vi "dfd_Filter Types Are All SOS.vi"(8 "error in (no error)":errorcluster, 11 "filters in":T1[](array[typedef]) {"mSRate_QSettings"."source" items=["Coef a/k"=0, "Coef b/v"=7, "Input"=1, "Output"=2, "Multiplicand"=3, "Product"=4, "Sum"=5, "Delay"=6, "Gain"=8]}) -> (0 "error out":errorcluster, 2 "All SOS?":bool, 3 "filters out":T1[](array[typedef]) {"mSRate_QSettings"."source" items=["Coef a/k"=0, "Coef b/v"=7, "Input"=1, "Output"=2, "Multiplicand"=3, "Product"=4, "Sum"=5, "Delay"=6, "Gain"=8]})   [LabVIEW 2017, in "NI_DigFilterLicensed.lvlib"]
uses:
  <vilib>/addons/Digital Filter Design/NI_DigFilterLicensed.lvlib
  <vilib>/addons/Digital Filter Design/_Objects.llb/DFD Filter Obj.ctl
  <vilib>/addons/Digital Filter Design/_Objects.llb/DFD Filter Coef.ctl
  <vilib>/addons/Digital Filter Design/_Objects.llb/DFD Filter Structure Type Selector.ctl
  <vilib>/addons/Digital Filter Design/_Objects.llb/dfd_Internal Quantization Settings.ctl
  <vilib>/addons/Digital Filter Design/_Objects.llb/dfd_Internal Quantization Srcs.ctl
  <vilib>/addons/Digital Filter Design/_Objects.llb/DFD Coef Norm Type.ctl
  <vilib>/addons/Digital Filter Design/_Objects.llb/DFD Filter Structure Id.ctl
  <vilib>/addons/Digital Filter Design/FilterLib.llb/dfd_Get Filter Coef Type (Filter IO).vi
  <vilib>/addons/Digital Filter Design/_Misc.llb/dfd_Error Handlers (Single).vi
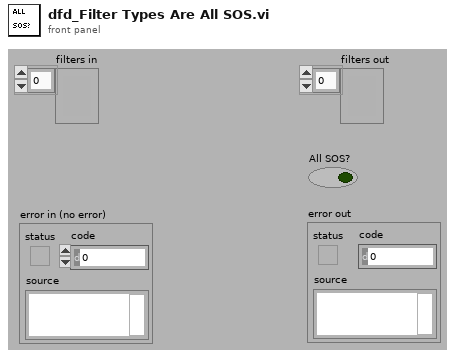
[diagram p1: front panel]
types:
  T1 = typedef "NI_DigFilterLicensed.lvlib/DFD Filter Obj.ctl" = cluster{"mSRate_Fs":dbl, "mSRate_Version":string, "mSRate_Comments":string, "mSRate_OrgCoef":T2, "mSRate_CurCoef":T2, "mSRate_Quantized?":bool, "mSRate_QCoef":T2, "mSRate_QSettings":T4[], "mSRate_Order":i32, "mSRate_Scaling":cluster{"mSRate_ScaleByPowerOf2?":bool, "mSRate_ScaleType":T6}}
  T2 = typedef "NI_DigFilterLicensed.lvlib/DFD Filter Coef.ctl" = cluster{"type":T3, "gain":dbl, "coef a (k)":dbl[], "coef b (v)":dbl[]}
  T3 = typedef "NI_DigFilterLicensed.lvlib/DFD Filter Structure Type Selector.ctl" = enum16{"Undefined", "FIR Direct Form", "FIR Direct Form Transposed", "FIR Symmetric", "FIR Antisymmetric", "IIR Direct Form I", "IIR Direct Form I Transposed", "IIR Direct Form II", "IIR Direct Form II Transposed", "IIR Cascaded Second Order Sections Form I", "IIR Cascaded Second Order Sections Form I Transposed", "IIR Cascaded Second Order Sections Form II", "IIR Cascaded Second Order Sections Form II Transposed", "Lattice Allpass (basic sections)", "Lattice Allpass (one multiplier sections)", "Lattice Allpass (normalized sections)", "Lattice AR (basic sections)", "Lattice AR (one multiplier sections)", "Lattice AR (normalized sections)", "Lattice MA (minimum phase)", "Lattice MA (maximum phase)", "Lattice ARMA (basic sections)", "Lattice ARMA (one multiplier sections)", "Lattice ARMA (normalized sections)"}
  T4 = typedef "NI_DigFilterLicensed.lvlib/dfd_Internal Quantization Settings.ctl" = cluster{"source":T5, "wl":i16, "iwl":i16, "overflow mode":enum16{"Saturation", "Wrap"}, "rounding mode":enum16{"Nearest", "Truncation"}, "signed?":bool}
  T5 = typedef "NI_DigFilterLicensed.lvlib/dfd_Internal Quantization Srcs.ctl" = u16
  T6 = typedef "NI_DigFilterLicensed.lvlib/DFD Coef Norm Type.ctl" = enum16{"No Norm", "Time Domain 1-Norm", "Time Domain 2-Norm", "Time Domain Inf-Norm"}
  T7 = typedef "NI_DigFilterLicensed.lvlib/DFD Filter Structure Id.ctl" = enum16{"Undefined", "FIR", "IIR Direct", "IIR SOS", "IIR Allpass", "IIR AR", "IIR ARMA"}
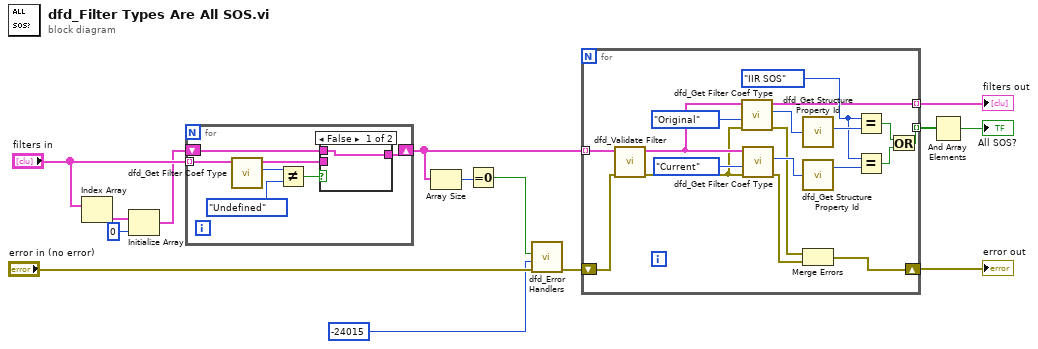
[diagram p0: block diagram]
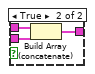
[diagram p2: hidden frame]
diagram:
  n1 = Index Array(array="filters in") -> (element=w8:T1)  [unwired: 1 in]
  n2 = Initialize Array(w8, 0 ("dimension size")) -> (w7:T1[])
  n3 = for {
    shift-right: [w19] -> w6
    shift-left: w7 -> [w18]
    tunnel: "filters in" -> [w17] mode=indexing
    n4 = call-poly <vilib>:"dfd_Get Filter Coef Type.vi"("filter in"=w17) -> ("type"=w21:T3, "filter out"=w16:T1)  [unwired: 2 in, 7 out]
    n5 = Not Equal?(x=w21, y=DFD_Filter_Structure_Type_Selector."Undefined") -> (x != y?=w15:bool)
    n6 = case shown="False" w15 {
      tunnel: [w22 w25] -> w19
      tunnel: w18 -> [w22 w24]
      tunnel: w16 -> [_ w23]
      frame False {
      }
      frame True {
        n7 = Build Array (concatenate)(w24, w23) -> (w25:T1[])
      }
    }
  }
  n8 = Array Size(array=w6) -> (size(s)=w5:i32)
  n9 = Equal To 0?(x=w5) -> (x = 0?=w2:bool)
  n10 = call-poly <vilib>:"dfd_Error Handlers.vi"("error in (no error)"="error in (no error)", "error code"=-24015 ("ERR_INVALID_FILTER_OBJ"), "condition failed?"=w2) -> ("error out"=w3:errorcluster)  [unwired: 8 out]
  n11 = for {
    tunnel: [w34] -> w11 mode=indexing
    shift-right: [w29] -> w14
    shift-left: w3 -> [w26]
    tunnel: [w28] -> w13 mode=indexing
    tunnel: w6 -> [w27] mode=indexing
    w37 = DFD_Filter_Structure_Id."IIR SOS" ("x")
    n12 = call <vilib>:"dfd_Validate Filter.vi"("error in (no error)"=w26, "filter in"=w27) -> ("error out"=w32:errorcluster, "filter out"=w33:T1)  [unwired: 1 in, 7 out]
    n13 = call-poly <vilib>:"dfd_Get Filter Coef Type.vi"("error in (no error)"=w32, "coef source"=enum16{"Original", "Current", "Quantized"}."Original", "filter in"=w33) -> ("error out"=w31:errorcluster, "type"=w41:T3, "filter out"=w28:T1)  [unwired: 6 out]
    n14 = call-poly <vilib>:"dfd_Get Filter Coef Type.vi"("error in (no error)"=w32, "coef source"=enum16{"Original", "Current", "Quantized"}."Current", "filter in"=w33) -> ("error out"=w30:errorcluster, "type"=w40:T3)  [unwired: 7 out]
    n15 = call <vilib>:"dfd_Get Structure Property Id.vi"("structure type"=w41) -> ("filter structure id"=w39:T7)  [unwired: 1 out]
    n16 = call <vilib>:"dfd_Get Structure Property Id.vi"("structure type"=w40) -> ("filter structure id"=w38:T7)  [unwired: 1 out]
    n17 = Merge Errors(w31, w30) -> (w29:errorcluster)
    n18 = Equal?(x=w37, y=w39) -> (x = y?=w36:bool)
    n19 = Equal?(x=w37, y=w38) -> (x = y?=w35:bool)
    n20 = Or(x=w36, y=w35) -> (x .or. y?=w34:bool)
  }
  "error out" <- w14
  "filters out" <- w13
  n21 = And Array Elements(Boolean array=w11) -> (logical AND=→"All SOS?":bool)
